vi "Send over UDP.vi"(1 "String to send":string, 2 "IP String":string="10.1.95.2") -> ()   [LabVIEW 2013]
panel:
  out "error out":errorcluster
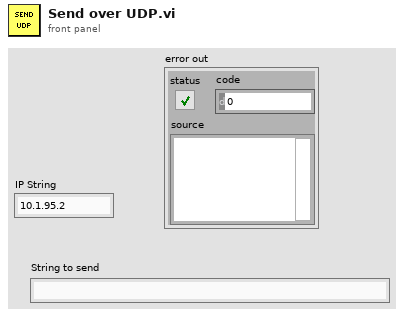
[diagram p1: front panel]
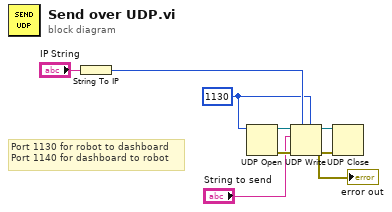
[diagram p0: block diagram]
diagram:
  w1 = u16 1130 ("port")
  # "Port 1130 for robot to dashboard\nPort 1140 for dashboard to robot"
  n1 = String To IP(1:"IP String") -> (0:w2:u32)
  n2 = UDP Open(11:w1) -> (port=w8:refnum<k16>, 0:w7:errorcluster)  [unwired: 4 in, 1 out]
  n3 = UDP Write(address=w2, port or service name=w1, connection ID=w8, data in="String to send", 8:w7) -> (error out=w6:errorcluster, 3:w5:refnum<k16>)  [unwired: 1 in]
  "error out" <- w6
  n4 = UDP Close(connection ID=w5, 8:w6) -> ()  [unwired: 2 out]
